vi "init.vi"(8 "error in (no error)":errorcluster, 11 "USB DAQ in":refnum<class "USB DAQ.lvclass">) -> (0 "error out":errorcluster, 3 "USB DAQ out":refnum<class "USB DAQ.lvclass">)   [LabVIEW 2025, in "USB DAQ.lvclass"]
uses:
  USB DAQ.lvclass
  USB DAQ.lvclass/USB DAQ.ctl
  Generic Handler/Generic Handler.lvclass
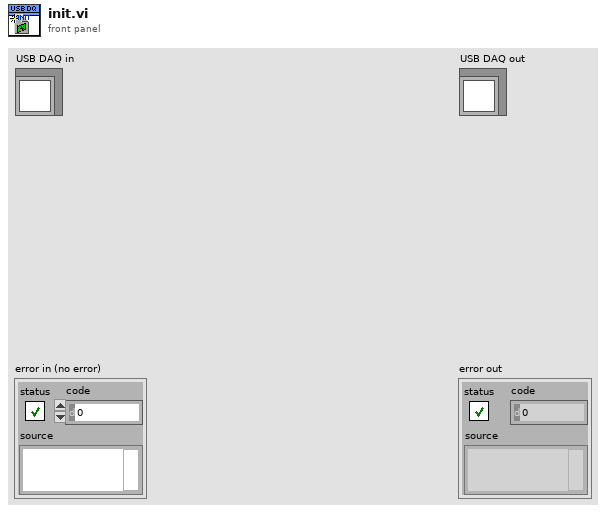
[diagram p1: front panel]
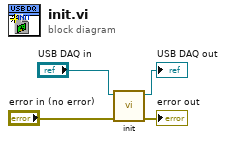
[diagram p0: block diagram]
diagram:
  n1 = call-parent "init.vi"("error in (no error)"="error in (no error)", "Generic Handler in"="USB DAQ in") -> ("error out"=→"error out":errorcluster, "Generic Handler out"=→"USB DAQ out":refnum<class "USB DAQ.lvclass">)  [unwired: 8 in]
